vi "4.4.1.vi"() -> ()   [LabVIEW 2018]
panel:
  out "배열":dbl[](array[numeric])
  out "숫자형":dbl
  out "결과":dbl
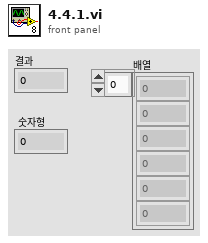
[diagram p1: front panel]
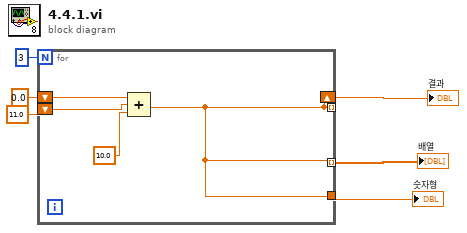
[diagram p0: block diagram]
diagram:
  n1 = for {
    N: 3 -> [_]
    shift-right: [w7] -> w5
    shift-left: 0.0 -> [w10]
    shift-left: 11.0 -> [w9]
    tunnel: [w7] -> _ mode=indexing
    tunnel: [w7] -> w1 mode=indexing
    tunnel: [w7] -> w2
    n2 = Compound Arithmetic op=ADD(w10, w9, 10.0 ("값")) -> (w7:dbl)
  }
  "결과" <- w5
  "숫자형" <- w2
  "배열" <- w1
